vi "Read Calibration Files.vi"(8 "Error In":errorcluster, 11 "LS218 in":refnum<class "LS218.lvclass">) -> (0 "Error Out":errorcluster, 3 "LS218 out":refnum<class "LS218.lvclass">)   [LabVIEW 2016, in "LS218.lvlib" / "LS218.lvclass"]
doc: "Read calibration files to be used from separate configuration."
uses:
  LS218.lvclass
  C:/User/Brand/LVP/STF/Packages/CSPP_Core/Actors/CS++BaseActor/CS++BaseActor.lvclass
  LS218.lvclass/LS218.ctl
  CSPP_Core/Actors/CS++BaseActor/CS++BaseActor.lvclass/CS++BaseActor.ctl
  <vilib>/Utility/config.llb/Read Key (String).vi
  CSPP_Core/Actors/CS++BaseActor/CS++BaseActor.lvclass
  <vilib>/Utility/config.llb/NI_LVConfig.lvlib
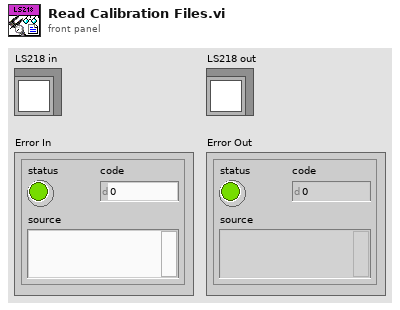
[diagram p1: front panel]
types:
  T1 = typedef "NI_LVConfig.lvlib/Config Data RefNum.ctl" = refnum<k1>
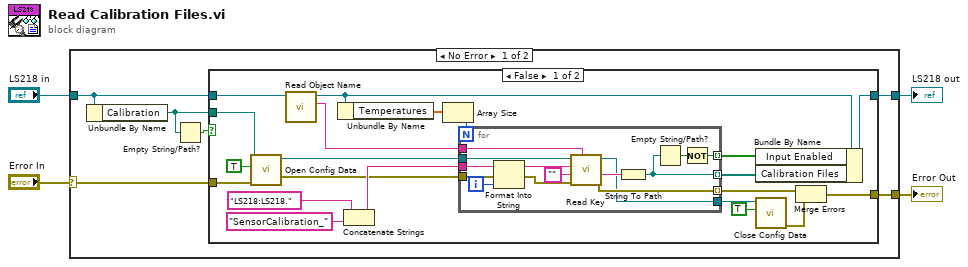
[diagram p0: block diagram]
diagram:
  n1 = case shown="No Error" "Error In" {
    selector: "Error In" -> [w10 w49]
    tunnel: [w7 w49] -> w3
    tunnel: [w8 w48] -> w1
    tunnel: "LS218 in" -> [w9 w48]
    frame No Error {
      n2 = Unbundle By Name(w9) -> ("Calibration"=w6:path)
      n3 = Empty String/Path?(string/path=w6) -> (empty?=w5:bool)
      n4 = case shown="False" w5 {
        tunnel: w6 -> [w19 _]
        tunnel: w10 -> [w17 w46]
        tunnel: w9 -> [w31 w47]
        tunnel: [w22 w47] -> w8
        tunnel: [w20 w46] -> w7
        frame False {
          n5 = call <vilib>:"Open Config Data.vi"("error in (no error)"=w17, "create file if necessary (T)"=TRUE, "configuration file path"=w19) -> ("error out"=w11:errorcluster, "refnum"=w15:T1)  [unwired: 6 in, 1 out]
          n6 = call "Read Object Name.vi"("CS++BaseActor in"=w31) -> ("Object Name"=w16:string, "CS++BaseActor out"=w23:refnum<class "LS218.lvclass">)  [unwired: 8 in, 1 out]
          n7 = Unbundle By Name(w23) -> ("Temperatures"=w27:dbl[unit][])
          n8 = Concatenate Strings("LS218:LS218.", "SensorCalibration_" ("string")) -> (w28:string)
          n9 = Array Size(array=w27) -> (size(s)=w26:i32)
          n10 = for {
            N: w26 -> [_]
            tunnel: w28 -> [w45]
            tunnel: w15 -> [w42]
            tunnel: [w39] -> w24 mode=indexing
            tunnel: [w37] -> w25 mode=indexing
            tunnel: w11 -> [w36]
            tunnel: [w34] -> w21 mode=indexing
            tunnel: w16 -> [w33]
            tunnel: [w32] -> w14
            i -> [w44]
            n11 = Format Into String(initial string=w45, error in=w36, w44) -> (resulting string=w43:string, error out=w35:errorcluster)  [unwired: 1 in]
            n12 = call-poly <vilib>:"Read Key.vi"("section"=w33, "error in (no error)"=w35, "default value"="", "key"=w43, "refnum"=w42) -> ("error out"=w34:errorcluster, "value"=w40:string, "refnum out"=w32:T1)  [unwired: 3 in, 1 out]
            n13 = String To Path(string=w40) -> (path=w39:path)
            n14 = Empty String/Path?(string/path=w39) -> (empty?=w38:bool)
            n15 = Not(x=w38) -> (.not. x?=w37:bool)
          }
          n16 = Bundle By Name(cluster=w23, "Input Enabled"=w25, "Calibration Files"=w24) -> (w22:refnum<class "LS218.lvclass">)
          n17 = call <vilib>:"Close Config Data.vi"("write file if changed (T)"=TRUE, "refnum"=w14) -> ("error out"=w12:errorcluster)  [unwired: 8 in, 1 out]
          n18 = Merge Errors(w21, w12) -> (w20:errorcluster)
        }
        frame True {
        }
      }
    }
    frame Error {
    }
  }
  "Error Out" <- w3
  "LS218 out" <- w1
